vi "Set Number of Samples.vi"(8 "error in (no error)":errorcluster, 9 "num samples":u64=1000, 10 "stream index":i32, 11 "refnum in":refnum<k20>) -> (0 "error out":errorcluster, 3 "refnum out":refnum<k20>)   [LabVIEW 2015, in "niInstr Streaming v1 Host.lvlib"]
doc: "This VI configures the number of samples to transfer when the stream is put into a finite transfer mode.\n\n<B>Input Parameters</B>\n\n<B>error in (no error)</B> 'error in' can accept error information wired from VIs previously called. Use this information to decide if any functionality should be bypassed in the event of errors from other VIs.\n\nRight-click the 'error in' control on the front panel and select 'Explain Error' or 'Explain Warning' from the shortcut menu for more information about the error.\n\n<B>stream index</B> Selects which stream index this VI will interface to. This is the index number at the end of the host interface controls (0..7).\n\n<B>Output Parameters</B>\n\n<B>error out</B> contains error information. This output provides standard error out functionality.\n\n<B>refnum out</B> Copy of refnum in"
uses:
  <instrlib>/_niInstr/Streaming/v1/Host/niInstr Streaming v1 Host.lvlib
  <instrlib>/_niInstr/Streaming/v1/Host/Public/Stream Host Interface.ctl
  <vilib>/rvi/errors/niLvFpgaAdjustHostInterfaceError.vi
  <vilib>/Utility/error.llb/Error Cluster From Error Code.vi
  <vilib>/rvi/interface/nirviReadWriteControl/nirviReadWriteControl.xnode
  <vilib>/ErrorRing/Error Ring.xnode
  NiFpgaLv.dll
  <vilib>/rvi/interface/Simulation/niFpgaSimulationCallBeginRW.vi
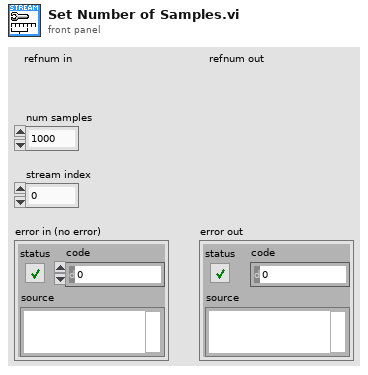
[diagram p1: front panel]
types:
  T1 = typedef "niInstr Streaming v1 Host.lvlib/Stream Host Interface.ctl" = refnum<k20>
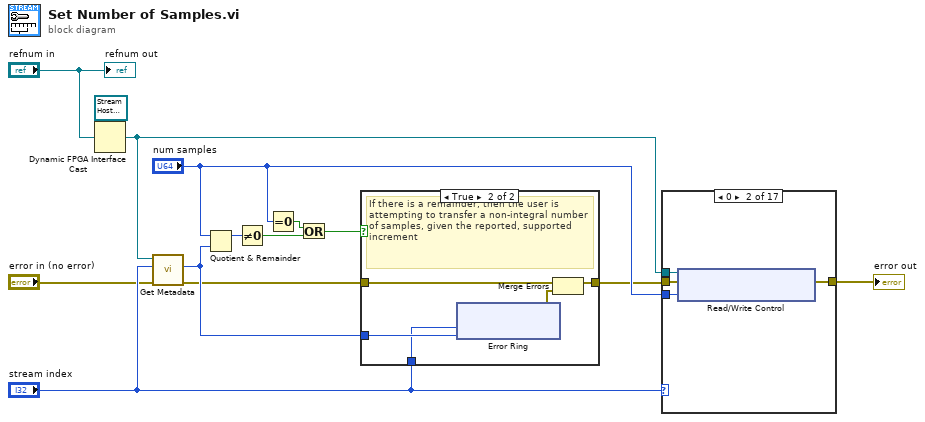
[diagram p0: block diagram]
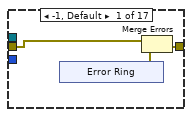
[diagram p3: hidden frame]
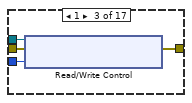
[diagram p4: hidden frame]
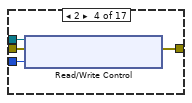
[diagram p5: hidden frame]
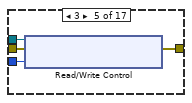
[diagram p6: hidden frame]
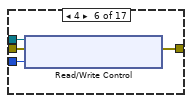
[diagram p7: hidden frame]
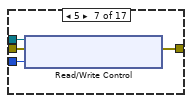
[diagram p8: hidden frame]
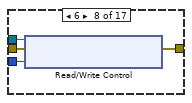
[diagram p9: hidden frame]
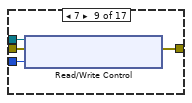
[diagram p10: hidden frame]
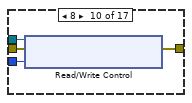
[diagram p11: hidden frame]
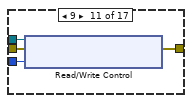
[diagram p12: hidden frame]
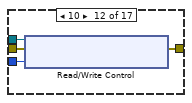
[diagram p13: hidden frame]
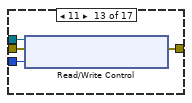
[diagram p14: hidden frame]
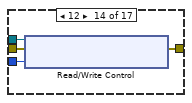
[diagram p15: hidden frame]
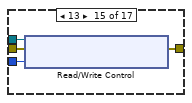
[diagram p16: hidden frame]
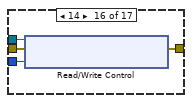
[diagram p17: hidden frame]
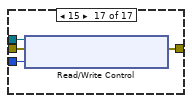
[diagram p18: hidden frame]
diagram:
  n1 = Dynamic FPGA Interface Cast(Session In=T1 refnum ("Refnum in"), Type="refnum in") -> (Session Out=w1:T1)
  n2 = call <instrlib>:"Get Metadata.vi"("error in (no error)"="error in (no error)", "stream index"="stream index", "refnum in"=w1) -> ("error out"=w5:errorcluster, "elements per cycle"=w8:u8)  [unwired: 6 in, 1 out]
  n3 = Quotient & Remainder(x="num samples", y=w8) -> (x-y*floor(x/y)=w12:u64)  [unwired: 1 out]
  n4 = Not Equal To 0?(x=w12) -> (x != 0?=w11:bool)
  n5 = Equal To 0?(x="num samples") -> (x = 0?=w14:bool)
  n6 = Or(x=w14, y=w11) -> (x .or. y?=w13:bool)
  n7 = case shown="False" w13 {
    tunnel: w5 -> [w15 w19]
    tunnel: [w15 w20] -> w6
    tunnel: w8 -> [_ w17]
    tunnel: "stream index" -> [_ w16]
    frame False {
    }
    frame True {
      # "If there is a remainder, then the user is attempting to transfer a non-integral number of samples, given the reported, supported increment"
      n8 = xnode "Error Ring"("parameter 0"=w16, "parameter 1"=w17) -> ("error out"=w18:errorcluster)
      n9 = Merge Errors(w19, w18) -> (w20:errorcluster)
    }
  }
  n10 = case shown="0" "stream index" {
    tunnel: w1 -> [_ w39 w43 w47 w51 w55 w59 w63 w67 w71 w75 w79 w83 w87 w91 w95 w99]
    tunnel: w6 -> [w29 w38 w42 w46 w50 w54 w58 w62 w66 w70 w74 w78 w82 w86 w90 w94 w98]
    tunnel: "num samples" -> [_ w37 w41 w45 w49 w53 w57 w61 w65 w69 w73 w77 w81 w85 w89 w93 w97]
    tunnel: [w30 w36 w40 w44 w48 w52 w56 w60 w64 w68 w72 w76 w80 w84 w88 w92 w96] -> w4
    frame -1, Default {
      n11 = xnode "Error Ring"() -> ("error out"=w31:errorcluster)
      n12 = Merge Errors(w29, w31) -> (w30:errorcluster)
    }
    frame 0 {
      n13 = xnode "Read/Write Control"("FPGA VI Reference In"=w39, "error in"=w38, "stream.num samples 0"=w37) -> ("error out"=w36:errorcluster)  [unwired: 1 out]
    }
    frame 1 {
      n14 = xnode "Read/Write Control"("FPGA VI Reference In"=w43, "error in"=w42, "stream.num samples 1"=w41) -> ("error out"=w40:errorcluster)  [unwired: 1 out]
    }
    frame 2 {
      n15 = xnode "Read/Write Control"("FPGA VI Reference In"=w47, "error in"=w46, "stream.num samples 2"=w45) -> ("error out"=w44:errorcluster)  [unwired: 1 out]
    }
    frame 3 {
      n16 = xnode "Read/Write Control"("FPGA VI Reference In"=w51, "error in"=w50, "stream.num samples 3"=w49) -> ("error out"=w48:errorcluster)  [unwired: 1 out]
    }
    frame 4 {
      n17 = xnode "Read/Write Control"("FPGA VI Reference In"=w55, "error in"=w54, "stream.num samples 4"=w53) -> ("error out"=w52:errorcluster)  [unwired: 1 out]
    }
    frame 5 {
      n18 = xnode "Read/Write Control"("FPGA VI Reference In"=w59, "error in"=w58, "stream.num samples 5"=w57) -> ("error out"=w56:errorcluster)  [unwired: 1 out]
    }
    frame 6 {
      n19 = xnode "Read/Write Control"("FPGA VI Reference In"=w63, "error in"=w62, "stream.num samples 6"=w61) -> ("error out"=w60:errorcluster)  [unwired: 1 out]
    }
    frame 7 {
      n20 = xnode "Read/Write Control"("FPGA VI Reference In"=w67, "error in"=w66, "stream.num samples 7"=w65) -> ("error out"=w64:errorcluster)  [unwired: 1 out]
    }
    frame 8 {
      n21 = xnode "Read/Write Control"("FPGA VI Reference In"=w71, "error in"=w70, "stream.num samples 8"=w69) -> ("error out"=w68:errorcluster)  [unwired: 1 out]
    }
    frame 9 {
      n22 = xnode "Read/Write Control"("FPGA VI Reference In"=w75, "error in"=w74, "stream.num samples 9"=w73) -> ("error out"=w72:errorcluster)  [unwired: 1 out]
    }
    frame 10 {
      n23 = xnode "Read/Write Control"("FPGA VI Reference In"=w79, "error in"=w78, "stream.num samples 10"=w77) -> ("error out"=w76:errorcluster)  [unwired: 1 out]
    }
    frame 11 {
      n24 = xnode "Read/Write Control"("FPGA VI Reference In"=w83, "error in"=w82, "stream.num samples 11"=w81) -> ("error out"=w80:errorcluster)  [unwired: 1 out]
    }
    frame 12 {
      n25 = xnode "Read/Write Control"("FPGA VI Reference In"=w87, "error in"=w86, "stream.num samples 12"=w85) -> ("error out"=w84:errorcluster)  [unwired: 1 out]
    }
    frame 13 {
      n26 = xnode "Read/Write Control"("FPGA VI Reference In"=w91, "error in"=w90, "stream.num samples 13"=w89) -> ("error out"=w88:errorcluster)  [unwired: 1 out]
    }
    frame 14 {
      n27 = xnode "Read/Write Control"("FPGA VI Reference In"=w95, "error in"=w94, "stream.num samples 14"=w93) -> ("error out"=w92:errorcluster)  [unwired: 1 out]
    }
    frame 15 {
      n28 = xnode "Read/Write Control"("FPGA VI Reference In"=w99, "error in"=w98, "stream.num samples 15"=w97) -> ("error out"=w96:errorcluster)  [unwired: 1 out]
    }
  }
  "error out" <- w4
  "refnum out" <- "refnum in"
